vi "SubVI_ProcessMeasName.vi"(9 "Write DAQ Size":u8, 10 "meas data type":T1 items=["UBYTE", "SBYTE", "UWORD", "SWORD", "ULONG", "SLONG", "FLOAT32_IEEE", "FLOAT64_IEEE", "A_UINT64", "A_INT64"], 11 "Meas Name":string) -> (1 "Meas Split Addr Offset":i32, 2 "Meas Split Flag":bool, 3 "DAQ List Signal Name":string[](array[string]))   [LabVIEW 2019, in "XCP_DaqDtoId.lvlib" / "DAQList.lvclass"]
uses:
  DAQList.lvclass
  <vilib>/ECUMC/ECUMC.llb/MC Data Type.ctt
  TypeDef/Global.vi
  <vilib>/ECUMC/ECUMC.lvlib
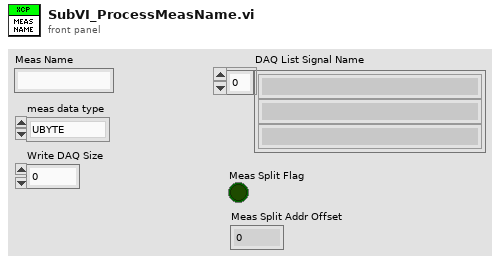
[diagram p1: front panel]
types:
  T1 = typedef "ECUMC.lvlib/MC Data Type.ctt" = u8
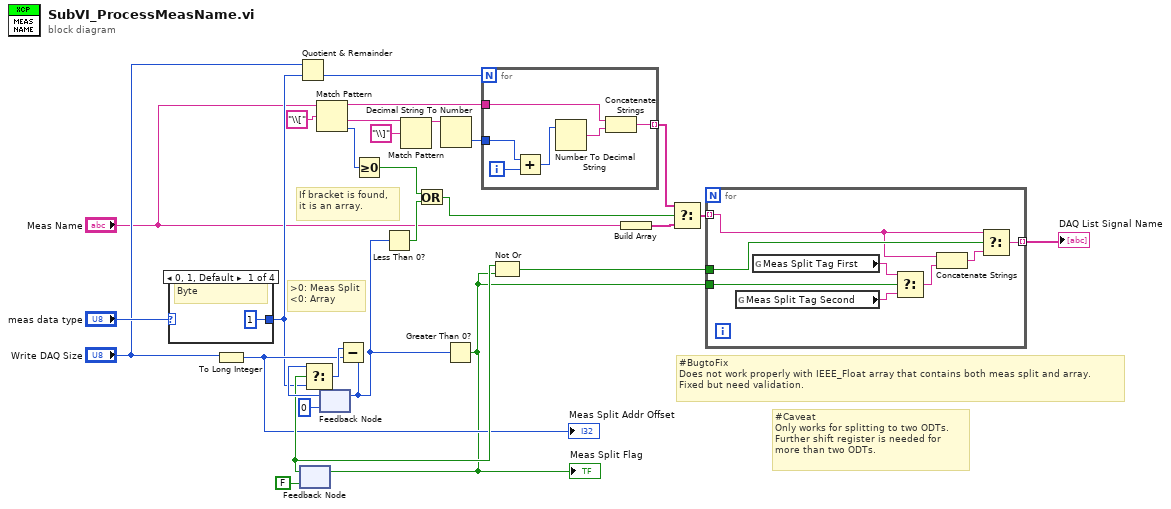
[diagram p0: block diagram]
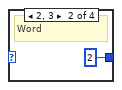
[diagram p2: hidden frame]
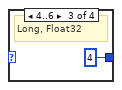
[diagram p3: hidden frame]
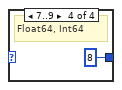
[diagram p4: hidden frame]
diagram:
  # "#BugtoFix\nDoes not work properly with IEEE_Float array that contains both meas split and array.\nFixed but need validation."
  # "If bracket is found, it is an array."
  # ">0: Meas Split\n<0: Array"
  # "#Caveat\nOnly works for splitting to two ODTs. Further shift register is needed for more than two ODTs."
  n1 = case shown="0, 1, Default" "meas data type" {
    tunnel: [1 2 4 8] -> w7
    frame 0, 1, Default {
      # "Byte"
    }
    frame 2, 3 {
      # "Word"
    }
    frame 4..6 {
      # "Long, Float32"
    }
    frame 7..9 {
      # "Float64, Int64"
    }
  }
  n2 = To Long Integer(number="Write DAQ Size") -> (32bit integer=w11:i32)
  "Meas Split Addr Offset" <- w11
  n3 = Quotient & Remainder(x="Write DAQ Size", y=w7) -> (floor(x/y)=w6:i32)  [unwired: 1 out]
  n4 = feedback #1(FALSE) -> (w26:bool)
  n5 = Match Pattern(string="Meas Name", regular expression="\\[") -> (before substring=w19:string, after substring=w22:string, offset past match=w15:i32)  [unwired: 1 in, 1 out]
  n6 = feedback #2(0) -> (w27:i32)
  n7 = Select(t=w27, s=w26, f=w7) -> (s? t:f=w28:i32)
  n8 = Subtract(x=w28, y=w11) -> (x-y=w25:i32)
  n9 = feedback-in #2(w25) -> ()
  n10 = Greater Or Equal To 0?(x=w15) -> (x >= 0?=w14:bool)
  n11 = Less Than 0?(x=w25) -> (x < 0?=w13:bool)
  n12 = Match Pattern(string=w22, regular expression="\\]") -> (before substring=w21:string)  [unwired: 1 in, 3 out]
  n13 = Or(x=w14, y=w13) -> (x .or. y?=w12:bool)
  n14 = Decimal String To Number(string=w21) -> (number=w18:i32)  [unwired: 2 in, 1 out]
  n15 = Greater Than 0?(x=w25) -> (x > 0?=w3:bool)
  "Meas Split Flag" <- w3
  n16 = feedback-in #1(w3) -> ()
  n17 = for {
    N: w6 -> [_]
    tunnel: w19 -> [w36]
    tunnel: w18 -> [w37]
    tunnel: [w34] -> w17 mode=indexing
    i -> [w38]
    n18 = Add(x=w37, y=w38) -> (x+y=w33:i32)
    n19 = Number To Decimal String(number=w33) -> (decimal integer string=w35:string)  [unwired: 1 in]
    n20 = Concatenate Strings(w36, w35) -> (w34:string)
  }
  n21 = Not Or(1:w3, 2:w26) -> (0:w2:bool)
  n22 = Build Array("Meas Name") -> (w16:string[])
  n23 = Select(t=w17, s=w12, f=w16) -> (s? t:f=w5:string[])
  n24 = for {
    tunnel: w5 -> [w40] mode=indexing
    tunnel: w3 -> [w42]
    tunnel: w2 -> [w41]
    tunnel: [w39] -> w1 mode=indexing
    n25 = global read "Global.vi" "Meas Split Tag Second"() -> (w46:string)
    n26 = global read "Global.vi" "Meas Split Tag First"() -> (w45:string)
    n27 = Select(t=w45, s=w42, f=w46) -> (s? t:f=w43:string)
    n28 = Concatenate Strings(w40, w43) -> (w44:string)
    n29 = Select(t=w40, s=w41, f=w44) -> (s? t:f=w39:string)
  }
  "DAQ List Signal Name" <- w1
